vi "trash_Write gRPC Server TS.vi"(8 "error in (no error)":errorcluster, 10 "gRPC Server":u64, 11 "CIFCorePlugin in":refnum<class "CIFCorePlugin.lvclass">) -> (0 "error out":errorcluster, 3 "CIFCorePlugin out":refnum<class "CIFCorePlugin.lvclass">)   [LabVIEW 2021]
doc: "Update the timestamp. Time is U64, absolute time in nS in the appropriate clockID configured for the plugin. If a 0 is wired it will automatically get the current time."
uses:
  CIFCorePlugin.lvclass
  CIFCorePlugin.lvclass/CIFCorePlugin.ctl
  CIFUtilities/CIFClocks/Time Conversion/LabVIEW Time to UTC Time.vi
  CIFUtilities/CIFClocks/SubVIs/Add Error.vi
  CIFUtilities/CIFClocks/CIFClocks.lvlib
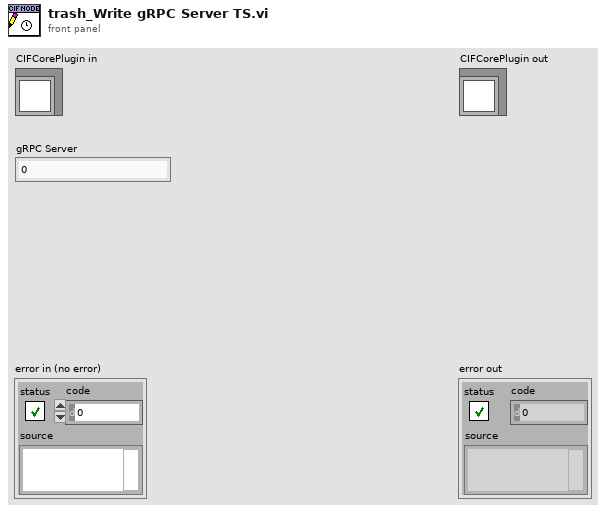
[diagram p1: front panel]
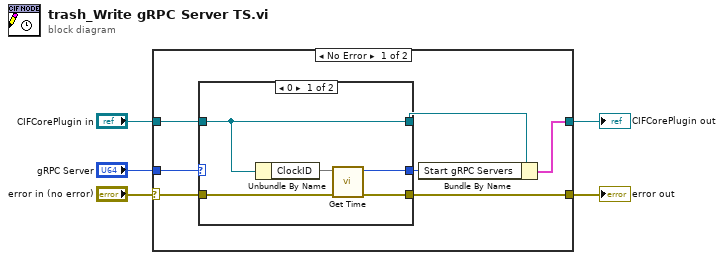
[diagram p0: block diagram]
diagram:
  n1 = case shown="No Error" "error in (no error)" {
    selector: "error in (no error)" -> [w10 w21]
    tunnel: [w6 w21] -> w4
    tunnel: [w12 w22] -> w2
    tunnel: "CIFCorePlugin in" -> [w9 w22]
    tunnel: "gRPC Server" -> [w11 _]
    frame No Error {
      n2 = case shown="0" w11 {
        selector: w11 -> [_ w19]
        tunnel: w10 -> [w15 w18]
        tunnel: w9 -> [w17 w20]
        tunnel: [w17 w20] -> w8
        tunnel: [w14 w19] -> w7
        tunnel: [w13 w18] -> w6
        frame 0 {
          n3 = Unbundle By Name(w17) -> ("ClockID"=w16)
          n4 = call "Get Time.vi"("error in (no error)"=w15, "ClockID"=w16) -> ("error out"=w13:errorcluster, "Time (ns)"=w14:u64)  [unwired: 7 in, 1 out]
        }
        frame 1, Default {
        }
      }
      n5 = Bundle By Name(cluster=w8, "Start gRPC Servers"=w7) -> (w12:cluster{})
    }
    frame Error {
    }
  }
  "error out" <- w4
  "CIFCorePlugin out" <- w2
